vi "Cancel Calibration.vi"(8 "error in (no error)":errorcluster, 10 "Boolean":bool, 11 "Queue in":refnum<queue>) -> (0 "error out":errorcluster, 2 "Cancel Calibration":bool)   [LabVIEW 2015]
uses:
  Message Queue/Message Cluster.ctl
  Message Queue/Enqueue Message (Single).vi
  Message Queue/Message Queue.lvlib
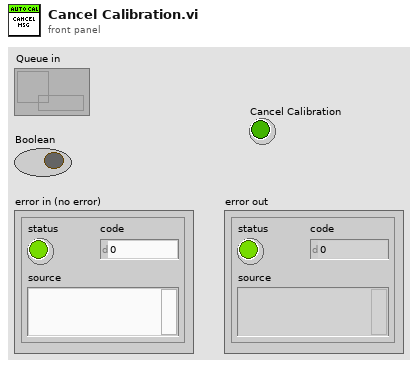
[diagram p1: front panel]
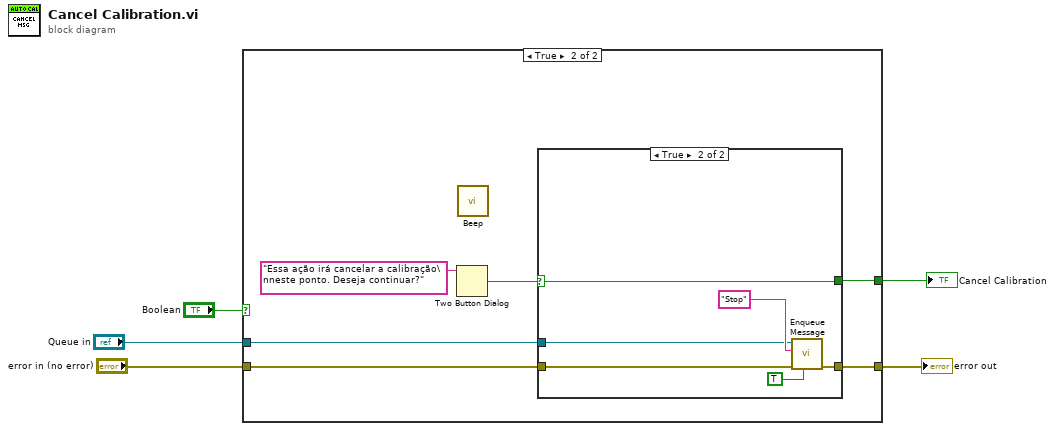
[diagram p0: block diagram]
diagram:
  n1 = case shown="True" "Boolean" {
    tunnel: "error in (no error)" -> [w6 w9]
    tunnel: "Queue in" -> [_ w8]
    tunnel: [w6 w10] -> w5
    tunnel: [_ w7] -> w1
    frame False {
    }
    frame True {
      n2 = Two Button Dialog(message="Essa ação irá cancelar a calibração\nneste ponto. Deseja continuar?") -> (T button?=w11:bool)  [unwired: 2 in]
      n3 = call <vilib>:"Beep.vi"() -> ()  [unwired: 12 in]
      n4 = case shown="True" w11 {
        selector: w11 -> [_ w14]
        tunnel: [w13 w18] -> w10
        tunnel: w9 -> [w13 w15]
        tunnel: w8 -> [_ w17]
        tunnel: [_ w14] -> w7
        frame False {
        }
        frame True {
          n5 = call-poly "Enqueue Message.vi"("Priority Message? (F)"=TRUE, "error in (no error)"=w15, "Message"="Stop", "Message Queue"=w17) -> ("error out"=w18:errorcluster)  [unwired: 6 in, 1 out]
        }
      }
    }
  }
  "error out" <- w5
  "Cancel Calibration" <- w1
